vi "2014 Target Detection.vi"(11 "Camera Image":T2(plugin-control)) -> (0 "Target Center (-1 to 1).X":dbl, 1 "Target Found":bool, 3 "Image":T2(plugin-control))   [LabVIEW 2013]
uses:
  TargetType.ctl
panel:
  in  "Color Components":T1={"Hue"={114.90465805469681, 184.83961478861238}, "Sat"={0.0, 255.0}, "Val"={170.0, 255.0}}
  in  "Score Cutoff":dbl=90.0 format="%#_13g"
  out "Distance (ft)":dbl
  in  "Instructions:":string="Images:\nUse the tab immediately below to choose the image source. Update the camera settings or the image directory so that you have images or video to test with.\n\nCalibration:\nYou can update Color Component ranges directly, or by clicking and drawing a line on the colored strip in the Image control. The Std Dev multipliers and where the strip is drawn determine the calibration values.\n\nUse Debugging tab to view the result of the color range threshold .\n\nArea Size LImit is used to ignore objects too small or far away to care about.\n\nThe Details tab contains score details for each target and subObject.\n\nCamera Type is used to select lens angles for distance calculation.\n\nVertical strips with no adjacent horizontal strip are identified as \"not hot\" and marked in blue.\nThe numeric scores indicate represent aspect ratio and rectangularity.\n\nWhen both strips are near enough, the pair is identified as \"hot\" and marked in green. Scores\nindicate the left, right, ratio of widths, and vertical positioning.\n\nAny score that falls below cutoff is drawn in red and bounding box is drawn in red."
  in  "Std Devs":cluster{"Hue":dbl, "Sat":dbl, "Val":dbl}={"Hue"=4.0, "Sat"=6.0, "Val"=4.0}
  in  "Camera Type":enum16{"206", "1011", "1013"}(ring)=enum."1013"
  in  "Tabbed Info":enum32{"Debugging", "Details"}(tab)
  out "Mask":T2(plugin-control)
  out "Target Info":T4(array[cluster])
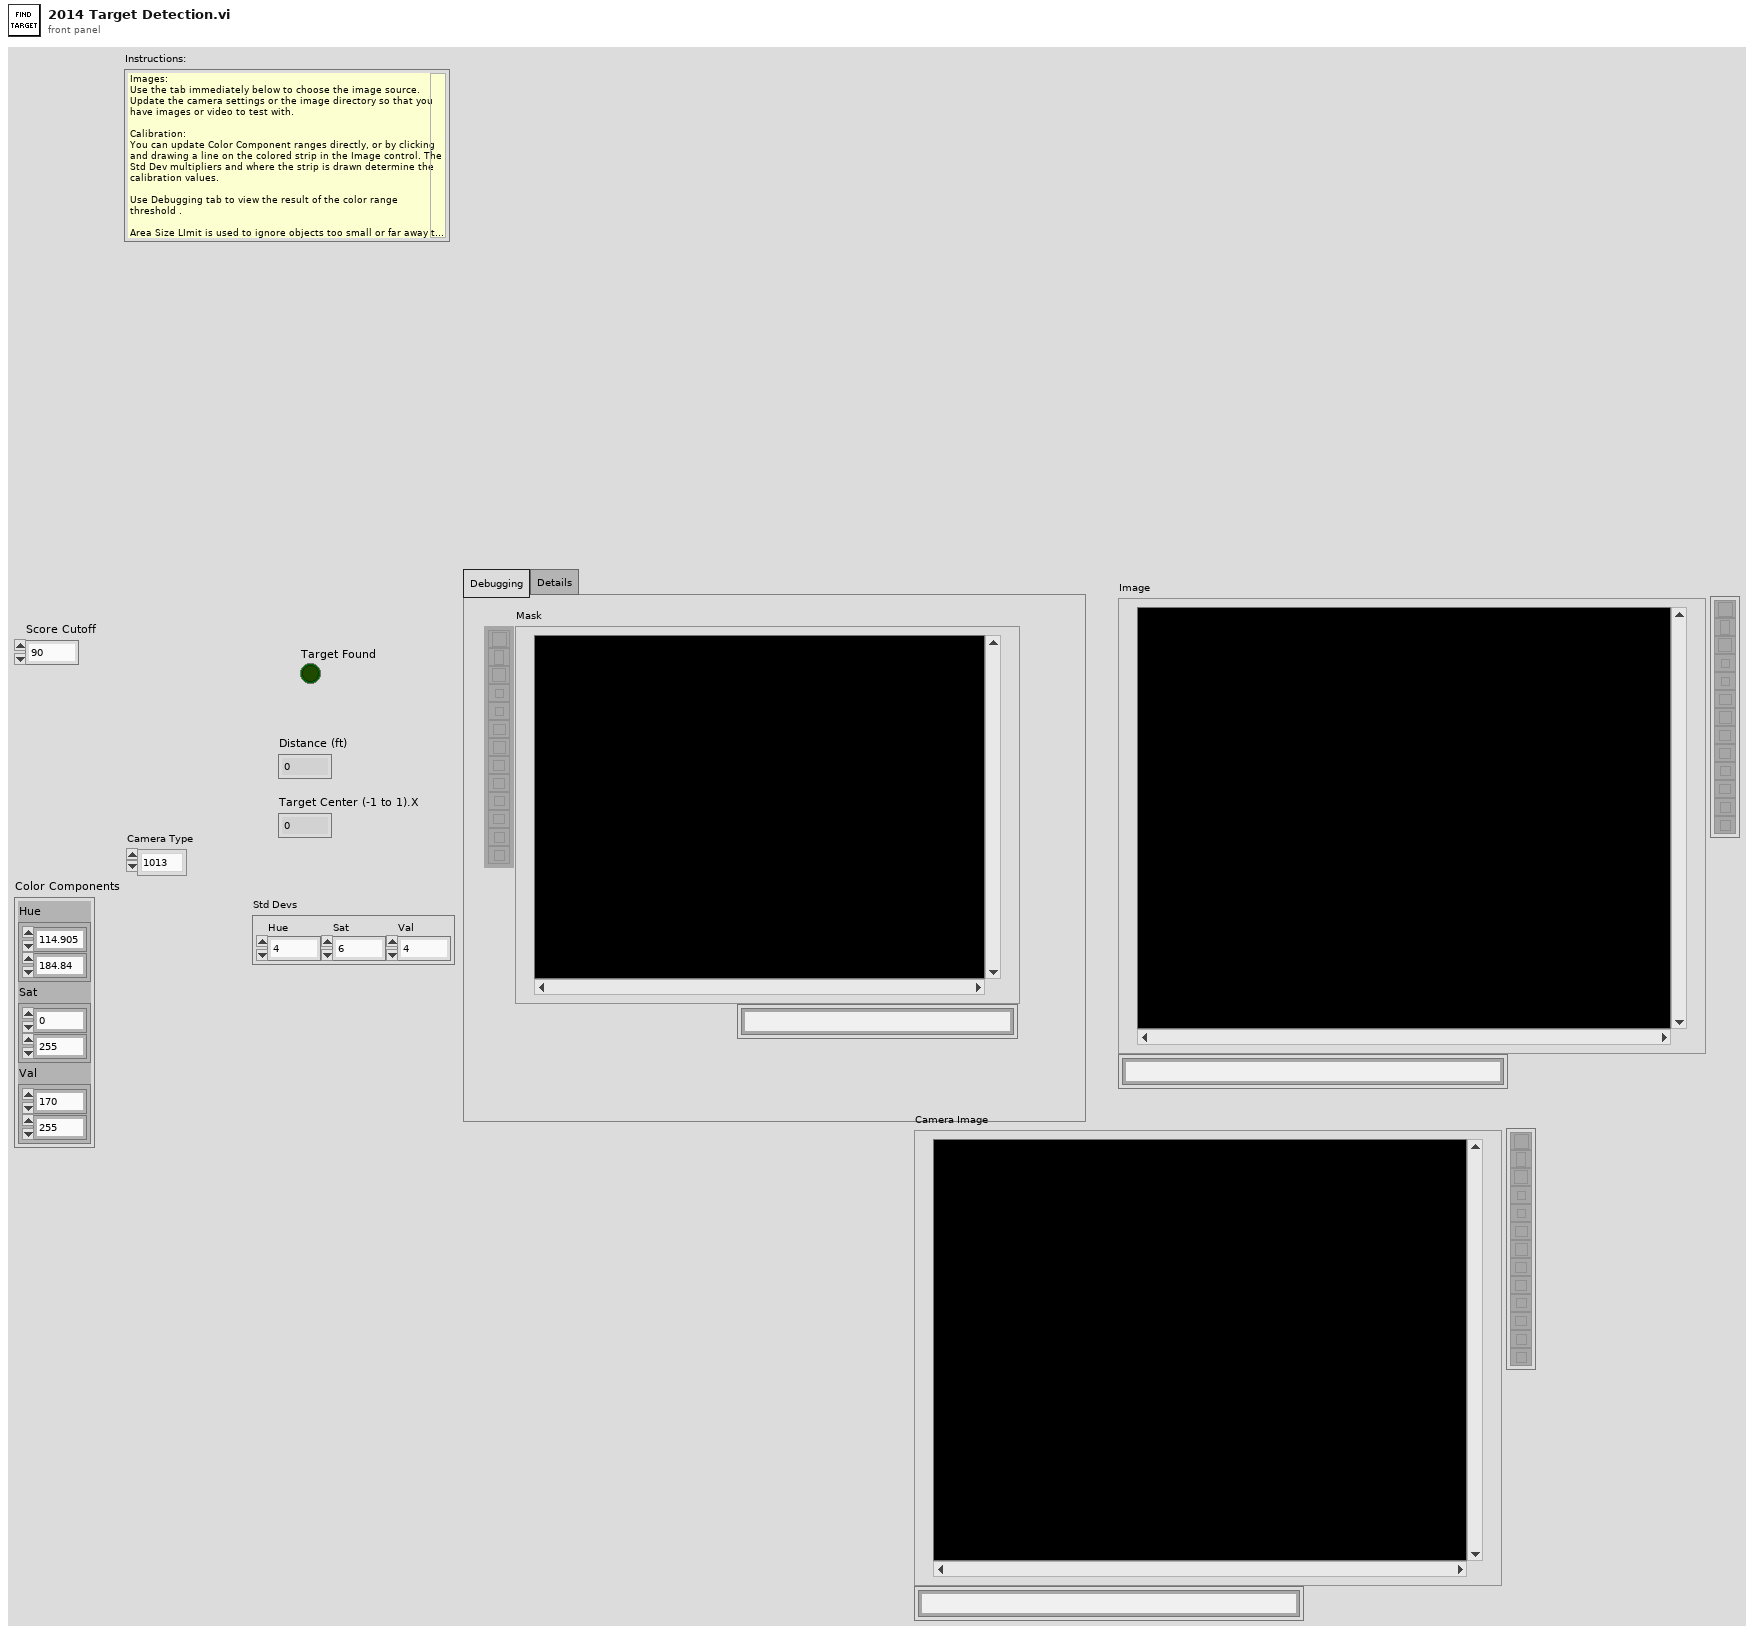
[diagram p1: front panel]
types:
  T1 = cluster{"Hue":cluster{dbl, dbl}, "Sat":cluster{dbl, dbl}, "Val":cluster{dbl, dbl}}
  T2 = typedef "IMAQ Image.ctl" = refnum<image>
  T3 = typedef "TargetType.ctl" = enum16{"Not Hot", "Hot"}
  T4 = cluster{"Scores":cluster{"Total":dbl, "Left":dbl, "Right":dbl, "Ratio":dbl, "Vertical":dbl, "index":i32, "State":T3}, "Verticals":cluster{"Horizontal?":bool, "Aspect Score":dbl, "Rect Score":dbl, cluster{"Left":dbl, "Top":dbl, "Right":dbl, "Bottom":dbl}, "Equiv H":dbl, "Equiv V":dbl}, "Horizontals":cluster{"Horizontal?":bool, "Aspect Score":dbl, "Rect Score":dbl, cluster{"Left":dbl, "Top":dbl, "Right":dbl, "Bottom":dbl}, "Equiv H":dbl, "Equiv V":dbl}, "Distance ft":dbl, "Center":cluster{"X":dbl, "Y":dbl}}[]
  T5 = typedef "Image Type" = u32
  T6 = cluster{"Horizontal":bool, "Aspect Score":dbl, "Rect Score":dbl, cluster{"Left":dbl, "Top":dbl, "Right":dbl, "Bottom":dbl}, "Equiv H":dbl, "Equiv V":dbl}[]
  T7 = cluster{"Scores":cluster{"Total":dbl, "Left":dbl, "Right":dbl, "Ratio":dbl, "Vertical":dbl, "index":i32, "State":T3}, "Verticals":cluster{"Horizontal?":bool, "Aspect Score":dbl, "Rect Score":dbl, cluster{"Left":dbl, "Top":dbl, "Right":dbl, "Bottom":dbl}, "Equiv H":dbl, "Equiv V":dbl}, "Horizontals":cluster{"Horizontal?":bool, "Aspect Score":dbl, "Rect Score":dbl, cluster{"Left":dbl, "Top":dbl, "Right":dbl, "Bottom":dbl}, "Equiv H":dbl, "Equiv V":dbl}, "Validated":bool}[]
  T8 = cluster{"Scores":cluster{"Total":dbl, "Left":dbl, "Right":dbl, "Ratio":dbl, "Vertical":dbl, "index":i32, "State":T3}, "Verticals":cluster{"Horizontal?":bool, "Aspect Score":dbl, "Rect Score":dbl, cluster{"Left":dbl, "Top":dbl, "Right":dbl, "Bottom":dbl}, "Equiv H":dbl, "Equiv V":dbl}, "Horizontals":cluster{"Horizontal?":bool, "Aspect Score":dbl, "Rect Score":dbl, cluster{"Left":dbl, "Top":dbl, "Right":dbl, "Bottom":dbl}, "Equiv H":dbl, "Equiv V":dbl}, "Distance (ft)":dbl, "Target Center (-1 to 1)":cluster{"X":dbl, "Y":dbl}}[]
  T9 = cluster{"Scores":cluster{"Total":dbl, "Left":dbl, "Right":dbl, "Ratio":dbl, "Vertical":dbl, "index":i32, "State":T3}, "Verticals":cluster{"Horizontal?":bool, "Aspect Score":dbl, "Rect Score":dbl, cluster{"Left":dbl, "Top":dbl, "Right":dbl, "Bottom":dbl}, "Equiv H":dbl, "Equiv V":dbl}, "Horizontals":cluster{"Horizontal?":bool, "Aspect Score":dbl, "Rect Score":dbl, cluster{"Left":dbl, "Top":dbl, "Right":dbl, "Bottom":dbl}, "Equiv H":dbl, "Equiv V":dbl}, "Distance (ft)":dbl, "Target Center (-1 to 1)":cluster{"X":dbl, "Y":dbl}}
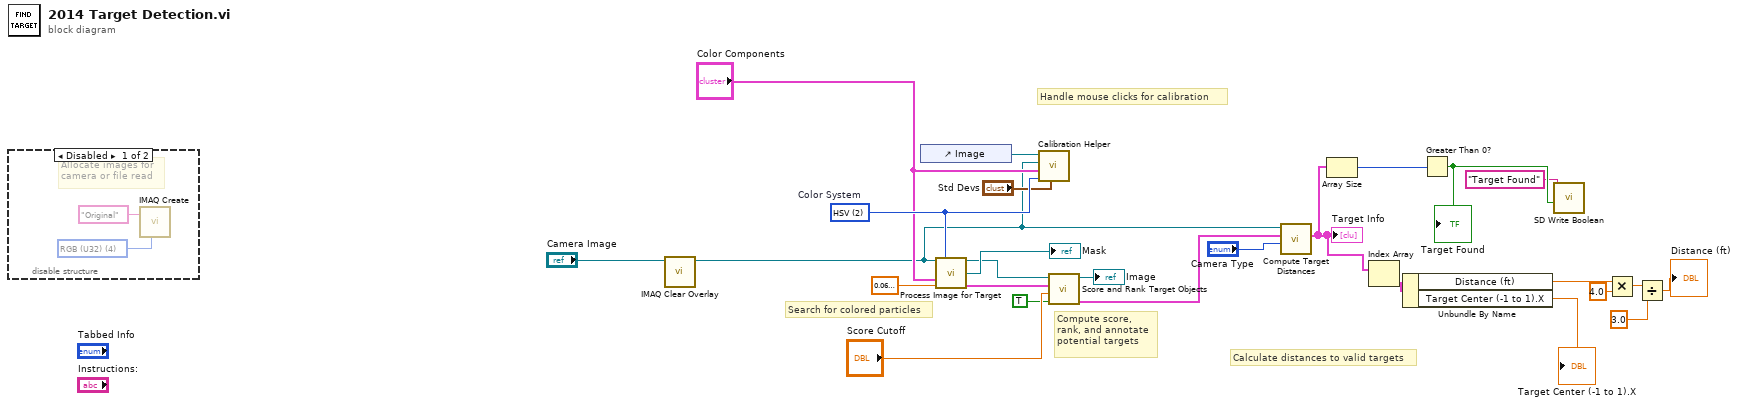
[diagram p0: block diagram]
diagram:
  w17 = u16 2 items=["RGB", "HSL", "HSV", "HSI"]  # Color System
  # "Calculate distances to valid targets"
  # "Search for colored particles"
  # "Handle mouse clicks for calibration"
  # "Compute score,\nrank, and annotate\npotential targets"
  n1 = disable-structure shown="Disabled" {
    frame Disabled {
      w28 = T5 4 items=["Grayscale (U8)", "Grayscale (I16)", "Grayscale (SGL)", "Complex (CSG)", "RGB (U32)", "HSL (U32)", "RGB (U64)", "Grayscale (U16)"] ("Image Type")
      # "Allocate images for\ncamera or file read"
      n2 = call "IMAQ Create"("Image Name"="Original", "Image Type"=w28) -> ()  [unwired: 3 in, 2 out]
    }
    frame Enabled {
    }
  }
  n3 = call "IMAQ Clear Overlay"("Image"="Camera Image") -> ("Image Out"=w14:T2)  [unwired: 9 in, 1 out]
  n4 = control-ref of="Image"() -> (w18:refnum<vi>)
  n5 = call "Process Image for Target.vi"("Src Image"=w14, "Color Mode"=w17, "Color Components"="Color Components", "Area Cutoff %"=0.06000000000000011 ("Area Size Limit %")) -> ("Src Image Out"=w24:T2, "Threshold"=→"Mask":T2, "Particles"=w21:T6)  [unwired: 9 in]
  n6 = call "Calibration Helper.vi"("Std Devs"="Std Devs", "Color Mode"=w17, "Color Components"="Color Components", "Image"=w14, "Image Ctl Refnum"=w18) -> ()  [unwired: 5 in, 2 out]
  n7 = call "Score and Rank Target Objects.vi"("Annotate"=TRUE, "Score Limit"="Score Cutoff", "Particles"=w21, "Image in"=w24) -> ("Target Info"=w20:T7, "Annotated Image"=→"Image":T2)  [unwired: 6 in]
  n8 = call "Compute Target Distances.vi"("Camera Type"="Camera Type", "Target Info"=w20, "Image in"=w14) -> ("Target Info"=w10:T8)  [unwired: 6 in, 2 out]
  "Target Info" <- w10
  n9 = Array Size(array=w10) -> (size(s)=w12:i32)
  n10 = Index Array(array=w10) -> (element=w9:T9)  [unwired: 1 in]
  n11 = Unbundle By Name(w9) -> ("Distance (ft)"=w8:dbl, "Target Center (-1 to 1).X"=→"Target Center (-1 to 1).X":dbl)
  n12 = Greater Than 0?(x=w12) -> (x > 0?=w2:bool)
  "Target Found" <- w2
  n13 = call <vilib>:"SD Write Boolean.vi"("Boolean"=w2, "Name"="Target Found") -> ()  [unwired: 8 in, 2 out]
  n14 = Multiply(x=w8, y=4.0) -> (x*y=w6:dbl)
  n15 = Divide(x=w6, y=3.0) -> (x/y=→"Distance (ft)":dbl)
